vi "Spartan Builder.vi"(8 "error in (no error)":errorcluster) -> (0 "error out":errorcluster)   [LabVIEW 2011]
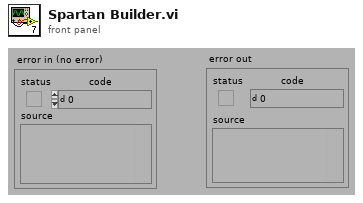
[diagram p1: front panel]
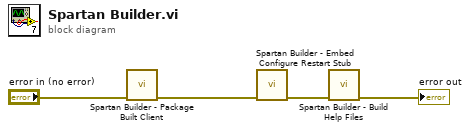
[diagram p0: block diagram]
diagram:
  n1 = call "Spartan Builder - Package Built Client.vi"("error in (no error)"="error in (no error)") -> ("error out"=w1:errorcluster)  [unwired: 10 out]
  n2 = call "Spartan Builder - Embed Configure Restart Stub.vi"("error in"=w1) -> ("error out"=w4:errorcluster)  [unwired: 10 out]
  n3 = call "Spartan Builder - Build Help Files.vi"("error in"=w4) -> ("error out"=→"error out":errorcluster)  [unwired: 10 out]
